vi "System Status Management.vi"(11 "CIFPluginManager in":refnum<class "CIFPluginManager.lvclass">) -> (0 "error out":errorcluster)   [LabVIEW 2021, in "CIFPluginManager.lvclass"]
uses:
  CIFPluginManager.lvclass
  CIFPluginManager.lvclass/CIFPluginManager.ctl
  CIFUtilities/CIFLogs/CIFLogs.lvlib
  gRPC/CIF_Manager_server/RPC Service/Manager/Manager.lvclass
  gRPC/CIF_Manager_server/RPC Messages/cif_manager_TimePair.ctl
  gRPC/CIF_Manager_server/CIF_Manager_server.lvlib
  gRPC/CIF_Manager_server/RPC Messages/cif_manager_ClockConversion.ctl
  gRPC/CIF_Manager_server/RPC Messages/cif_manager_ClockConversionArray.ctl
  gRPC/CIF_Manager_server/RPC Messages/cif_manager_SystemStatus.ctl
  <vilib>/CIF Foundation/CIF Utilities/Time/Time_CIF_U.lvlib
  gRPC/CIF_Manager_Client_Wrapper/CIFManagerClientWrapper.lvlib
  C:/Program Files/National Instruments/LabVIEW 2021/vi.lib/gRPC/LabVIEW gRPC Servicer/ServiceBase/ServiceBase.lvclass
  D:/dev/CIF-LVCore/src/CIFPluginManager/CIFPluginManager/gRPC/CIF_Manager_server/RPC Service/Manager/Manager.lvclass
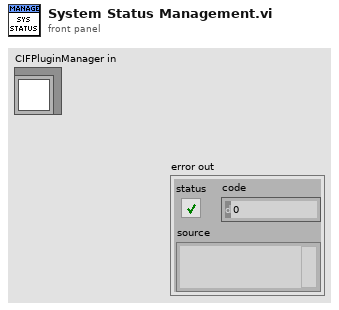
[diagram p1: front panel]
types:
  T1 = typedef "CIF_Manager_server.lvlib/Manager.lvclass/Server gRPC UEs.ctl" = cluster{"Manager LoadPlugin gRPC UE":refnum<user-event>, "Manager RegisterPlugin gRPC UE":refnum<user-event>, "Manager UnregisterPlugin gRPC UE":refnum<user-event>, "Manager QueryPluginTypes gRPC UE":refnum<user-event>, "Manager AbortPlugin gRPC UE":refnum<user-event>, "Manager UnloadAllPlugins gRPC UE":refnum<user-event>, "Manager Destroy gRPC UE":refnum<user-event>, "Manager Ping gRPC UE":refnum<user-event>, "Manager QueryErrors gRPC UE":refnum<user-event>, "Manager QueryConfig gRPC UE":refnum<user-event>, "Manager QueryInfo gRPC UE":refnum<user-event>, "Manager ResetErrorIndex gRPC UE":refnum<user-event>, "Manager ResetConfigIndex gRPC UE":refnum<user-event>, "Manager ResetInfoIndex gRPC UE":refnum<user-event>, "Manager QueryPluginInfo gRPC UE":refnum<user-event>, "Manager QueryPlugin gRPC UE":refnum<user-event>, "Manager QuerySystemStatus gRPC UE":refnum<user-event>, "Manager UpdateClock gRPC UE":refnum<user-event>, "Manager CreateOrch gRPC UE":refnum<user-event>, "Manager QueryClockStatus gRPC UE":refnum<user-event>, "Manager QueryAllChannels gRPC UE":refnum<user-event>, "Manager RegisterLauncher gRPC UE":refnum<user-event>, "Manager CreateLauncher gRPC UE":refnum<user-event>, "Manager DestroyLauncher gRPC UE":refnum<user-event>}
  T2 = typedef "CIF_Manager_server.lvlib/cif_manager_SystemStatus.ctl" = cluster{"clock_conversion_array":T3}
  T3 = typedef "CIF_Manager_server.lvlib/cif_manager_ClockConversionArray.ctl" = cluster{"clock_conversions":T4[]}
  T4 = typedef "CIF_Manager_server.lvlib/cif_manager_ClockConversion.ctl" = cluster{"clock_id":u32, "last_reset":i64, "slope":dbl, "offset_pair":T5, "clock_name":string}
  T5 = typedef "CIF_Manager_server.lvlib/cif_manager_TimePair.ctl" = cluster{"system_time":i64, "external_time":i64}
  T6 = typedef "grpc-lvsupport-release.lvlib/grpcId.ctl" = u64
  T7 = typedef "CIF_Manager_server.lvlib/cif_manager_PluginStatus.ctl" = cluster{"pluginname":T8, "status":T9, "channels":T18}
  T8 = typedef "CIF_Manager_server.lvlib/cif_manager_PluginName.ctl" = cluster{"plugin_name":string}
  T9 = typedef "CIF_Manager_server.lvlib/cif_plugincore_StatusData.ctl" = cluster{"state":T10, "timing_statistics":T11, "fifo_statistics":T13, "error":T14, "monitor_doubles":T15, "monitor_u64s":T16, "monitor_i64s":T17}
  T10 = typedef "CIF_Manager_server.lvlib/cif_plugincore_StatusData_PluginState.ctl" = enum32{"PLUGINSTATE_UNKNOWN", "PLUGINSTATE_CREATING", "PLUGINSTATE_LISTENING", "PLUGINSTATE_RUNNING", "PLUGINSTATE_CLEANINGUP", "PLUGINSTATE_DESTROYING"}
  T11 = typedef "CIF_Manager_server.lvlib/cif_plugincore_TimingStatistics.ctl" = cluster{"period":T12, "wake_error":T12, "execute":T12, "housekeep":T12, "idle":T12, "cleanup":T12, "custom_1":T12, "custom_2":T12}
  T12 = typedef "CIF_Manager_server.lvlib/cif_common_TimingStats.ctl" = cluster{"max":i64, "min":i64, "avg":dbl}
  T13 = typedef "CIF_Manager_server.lvlib/cif_plugincore_FifoStatistics.ctl" = cluster{"from_t0":T12, "from_previous_plugin":T12, "output_error":T12}
  T14 = typedef "CIF_Manager_server.lvlib/cif_plugincore_Error.ctl" = cluster{"status":bool, "code":i32}
  T15 = typedef "CIF_Manager_server.lvlib/cif_plugincore_MonitorDoubles.ctl" = cluster{"double_1":dbl, "double_2":dbl, "double_3":dbl, "double_4":dbl}
  T16 = typedef "CIF_Manager_server.lvlib/cif_plugincore_MonitorU64.ctl" = cluster{"u64_1":u64, "u64_2":u64, "u64_3":u64, "u64_4":u64}
  T17 = typedef "CIF_Manager_server.lvlib/cif_plugincore_MonitorI64.ctl" = cluster{"i64_1":i64, "i64_2":i64, "i64_3":i64, "i64_4":i64}
  T18 = typedef "CIF_Manager_server.lvlib/cif_channelcore_Channels.ctl" = cluster{"channels":T19[]}
  T19 = typedef "CIF_Manager_server.lvlib/cif_channelcore_Channel.ctl" = cluster{"name":string, "direction":T20, "type":string, "custom_config":u8[], "connected":bool, "connected_name":string, "forced":bool, "channel_pattern":T21}
  T20 = typedef "CIF_Manager_server.lvlib/cif_channelcore_ChannelDirection.ctl" = enum32{"CHANNELDIRECTION_UNKNOWN", "CHANNELDIRECTION_PUBLISHER", "CHANNELDIRECTION_SUBSCRIBER"}
  T21 = typedef "CIF_Manager_server.lvlib/cif_channelcore_ChannelPattern.ctl" = enum32{"CHANNELPATTERN_UNKNOWN", "CHANNELPATTERN_TAG", "CHANNELPATTERN_FIFO", "CHANNELPATTERN_MULTIFIFO", "CHANNELPATTERN_BACKPRESSUREFIFO"}
  T22 = typedef "Time_CIF_U.lvlib/Clock History Map.ctl" = map{u8, T23}
  T23 = typedef "Time_CIF_U.lvlib/Clock History.ctl" = cluster{"System Clock":i64[], "External Clock":i64[], "Last Reset Time":i64, "slope":dbl, "1/slope":dbl, "Offset Pair":T24, "Name":string}
  T24 = typedef "Time_CIF_U.lvlib/Timestamp Pair.ctl" = cluster{"System Time":i64, "External Time":i64}
  T25 = typedef "Time_CIF_U.lvlib/Clock Conversion.ctl" = cluster{"ClockID":u8, "Last Reset":i64, "Offset Pair":T24, "Slope":dbl, "1/Slope":dbl, "Name":string}
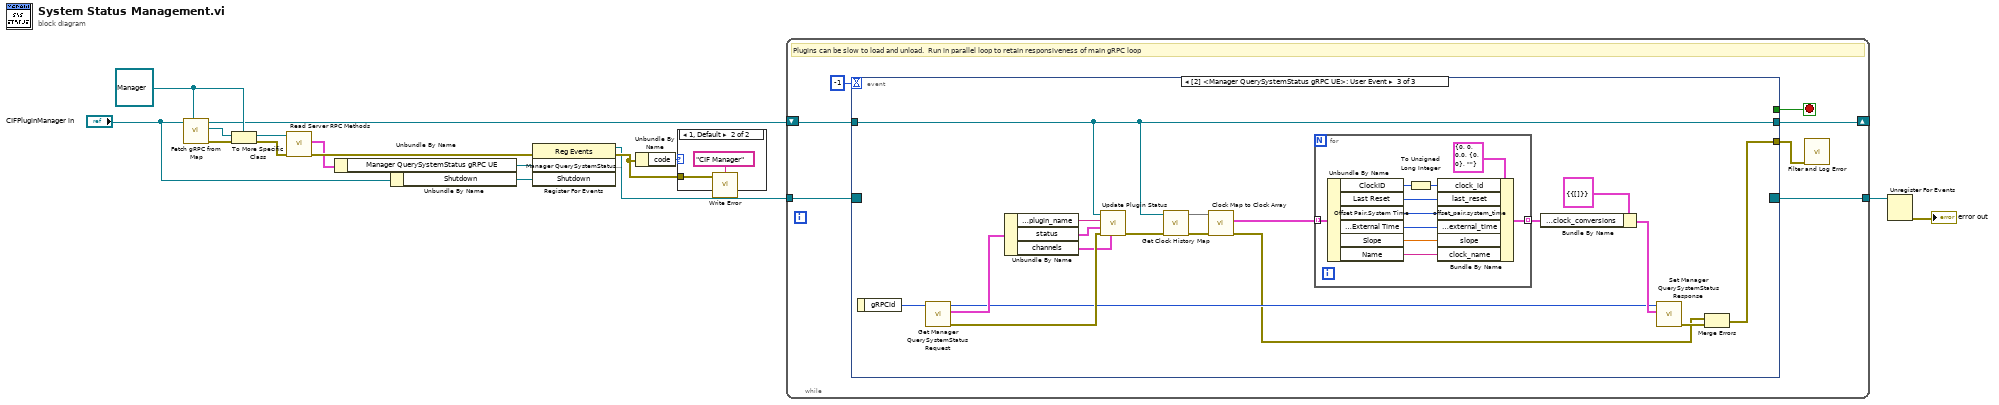
[diagram p0: block diagram]
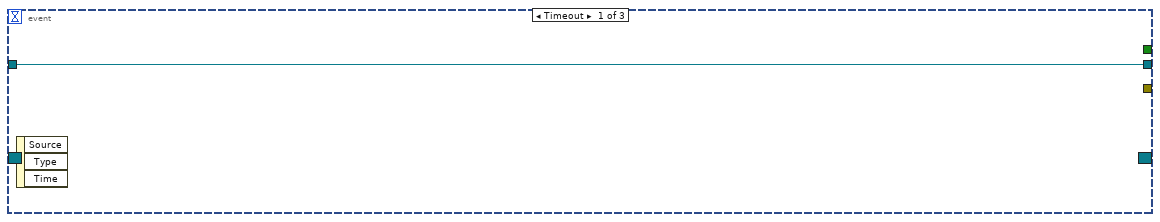
[diagram p3: hidden frame]
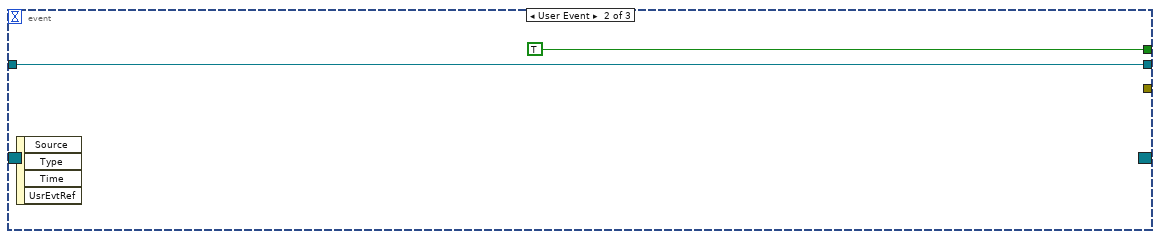
[diagram p4: hidden frame]
diagram:
  w12 = refnum<class "Manager.lvclass"> refnum ("CIF_Manager_server.lvlib:Manager.lvclass")
  n1 = call "Fetch gRPC from Map.vi"("gRPC Server Class type"=w12, "Plugin Manager in"="CIFPluginManager in") -> ("error out"=w11:errorcluster, "gRPC Server Class out"=w13:refnum<class "ServiceBase.lvclass">, "Plugin Manager out"=w4:refnum<class "CIFPluginManager.lvclass">)  [unwired: 7 in]
  n2 = To More Specific Class(target class=w12, reference=w13, error in=w11) -> (specific class reference=w9:refnum<class "Manager.lvclass">, error out=w10:errorcluster)
  n3 = call "Read Server RPC Methods.vi"("error in (no error)"=w10, "SignalGeneratorService in"=w9) -> ("error out"=w3:errorcluster, "Server RPC Methods"=w2:T1)  [unwired: 7 in, 1 out]
  n4 = Unbundle By Name(w2) -> ("Manager QuerySystemStatus gRPC UE"=w1:refnum<user-event>)
  n5 = Unbundle By Name("CIFPluginManager in") -> ("Shutdown"=w8:refnum<user-event>)
  n6 = register-events(error in=w3, w1, w8) -> (reference out=w5:refnum<event-registration>, error out=w6:errorcluster)  [unwired: 1 in]
  n7 = Unbundle By Name(w6) -> ("code"=w14:i32)
  n8 = case shown="1, Default" w14 {
    tunnel: w6 -> [_ w18]
    frame 0 {
      # "-1001 is cancelled by client.  Not an error."
    }
    frame 1, Default {
      n9 = call "Write Error.vi"("error in (no error)"=w18, "Plugin Name"="CIF Manager") -> ()  [unwired: 2 in, 1 out]
    }
  }
  n10 = while {
    tunnel: w5 -> [w25]
    shift-right: [w20] -> _
    shift-left: w4 -> [w24]
    tunnel: [w21] -> w15
    stop <- w22 stop-if-true
    # "Plugins can be slow to load and unload.  Run in parallel loop to retain responsiveness of main gRPC loop"
    n11 = event shown="[2] <Manager QuerySystemStatus gRPC UE>: User Event" {
      selector: w25 -> [_ _ _]
      dyn-events: [_ _ _] -> w21
      timeout: -1 -> [_ _ _]
      tunnel: w24 -> [w26 w27 w30]
      tunnel: [_ TRUE _] -> w22
      tunnel: [_ _ w35] -> w19
      tunnel: [w26 w27 w30] -> w20
      event Timeout {
        n12 = event-data() -> ()  [unwired: 1 in, 3 out]
      }
      event User Event {
        n13 = event-data() -> ()  [unwired: 1 in, 4 out]
      }
      event User Event {
        n14 = event-data() -> ("gRPCid"=w36:T6)  [unwired: 1 in]
        n15 = call "Get Manager QuerySystemStatus Request.vi"("gRPCid"=w36) -> ("error out"=w45:errorcluster, "Message Data"=w42:T7, "gRPCid out"=w38:T6)  [unwired: 8 in]
        n16 = Unbundle By Name(w42) -> ("pluginname.plugin_name"=w43:string, "status"=w44:T9, "channels"=w29:T18)
        n17 = call "Update Plugin Status.vi"("channels"=w29, "error in (no error)"=w45, "Status"=w44, "Plugin Name"=w43, "Launcher in"=w30) -> ("error out"=w33:errorcluster)  [unwired: 6 in]
        n18 = call "Get Clock History Map.vi"("error in (no error)"=w33, "CIFPluginManager in"=w30) -> ("error out"=w32:errorcluster, "Clock History Map"=w34:T22)  [unwired: 8 in]
        n19 = call <vilib>:"Clock Map to Clock Array.vi"("error in (no error)"=w32, "Clock History Map in"=w34) -> ("error out"=w31:errorcluster, "Clock Conversion Array"=w46:T25[])  [unwired: 7 in, 1 out]
        n20 = for {
          tunnel: w46 -> [w55] mode=indexing
          tunnel: [w47] -> w40 mode=indexing
          n21 = Unbundle By Name(w55) -> ("ClockID"=w54:u8, "Last Reset"=w48:i64, "Offset Pair.System Time"=w49:i64, "Offset Pair.External Time"=w50:i64, "Slope"=w51:dbl, "Name"=w52:string)
          n22 = To Unsigned Long Integer(number=w54) -> (unsigned 32bit integer=w53:u32)
          n23 = Bundle By Name(cluster=T4 {"clock_id"=0, "last_reset"=0, "slope"=0.0, "offset_pair"={"system_time"=0, "external_time"=0}, "clock_name"=""} ("cif_manager_ClockConversion"), "clock_id"=w53, "last_reset"=w48, "offset_pair.system_time"=w49, "offset_pair.external_time"=w50, "slope"=w51, "clock_name"=w52) -> (w47:T4)
        }
        n24 = Bundle By Name(cluster=T2 {"clock_conversion_array"={"clock_conversions"=[]}} ("Message Data"), "clock_conversion_array.clock_conversions"=w40) -> (w41:T2)
        n25 = call "Set Manager QuerySystemStatus Response.vi"("Message Data"=w41, "gRPCid in"=w38) -> ("error out"=w39:errorcluster)  [unwired: 9 in]
        n26 = Merge Errors(w31, w39) -> (w35:errorcluster)
      }
    }
    n27 = call "Filter and Log Error.vi"("error In"=w19) -> ()  [unwired: 11 in]
  }
  n28 = Unregister For Events(event registration refnum=w15) -> (error out=→"error out":errorcluster)  [unwired: 1 in]
